vi "SP Stimulus Debuging Tool.vi"(5 "New Stimulus":T1={"Use Instrument Settings"=FALSE, "Blank Frequencies"=FALSE, "Sweep Type"=enum."Linear", "Sweep"={"Fstart"=500.0, "Fstop"=1500.0, "Units"=enum."MHz", "Points"=201}, "Power (dBm)"=999.0, "IFBW (Hz)"=-1.0, "Sweep Time (s)"=-1.0, "Calibration"={"State"=FALSE, "String"=""}} {"Sweep Time (s)" format="%.3g"}, 7 "Current Stimulus":T1={"Use Instrument Settings"=FALSE, "Blank Frequencies"=FALSE, "Sweep Type"=enum."Linear", "Sweep"={"Fstart"=500.0, "Fstop"=1500.0, "Units"=enum."MHz", "Points"=201}, "Power (dBm)"=999.0, "IFBW (Hz)"=-1.0, "Sweep Time (s)"=-1.0, "Calibration"={"State"=FALSE, "String"=""}} {"Sweep Time (s)" format="%.3g"}, 8 "Overall":bool, 9 "SweepTime":bool, 10 "IFBW":bool, 11 "Power":bool) -> ()   [LabVIEW 2011]
uses:
  TypeDefs/SP Stimulus Parameters.ctl
  TypeDefs/SP Frequency Units.ctl
  TypeDefs/SP Calibration State.ctl
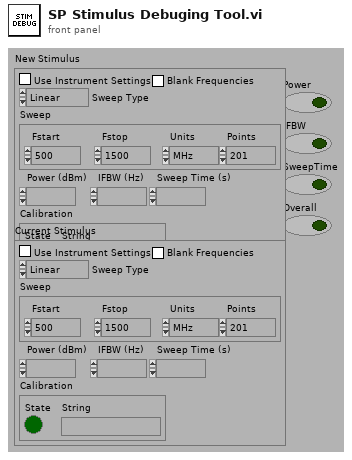
[diagram p1: front panel]
types:
  T1 = typedef "SP Stimulus Parameters.ctl" = cluster{"Use Instrument Settings":bool, "Blank Frequencies":bool, "Sweep Type":enum32{"Linear", "Logarithmic", "List", "Power", "CW"}, "Sweep":cluster{"Fstart":dbl, "Fstop":dbl, "Units":T2, "Points":i32}, "Power (dBm)":dbl, "IFBW (Hz)":dbl, "Sweep Time (s)":dbl, "Calibration":T3}
  T2 = typedef "SP Frequency Units.ctl" = enum16{"Hz", "kHz", "MHz", "GHz", "Points"}
  T3 = typedef "SP Calibration State.ctl" = cluster{"State":bool, "String":string}
  T4 = cluster{"Fstart":dbl, "Fstop":dbl, "Units":T2, "Points":i32}
  T5 = enum32{"Linear", "Logarithmic", "List", "Power", "CW"}
  T6 = enum32{"invalid app kind", "Development System", "Run Time System", "Student Edition", "Embedded LabVIEW", "Evaluation", "Custom"}
  T7 = enum16{"open", "replace", "create", "open or create", "replace or create", "replace or create with confirmation"}
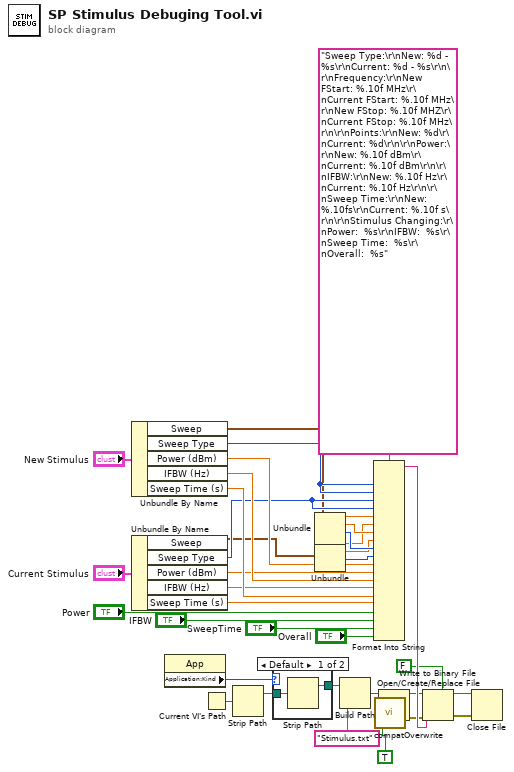
[diagram p0: block diagram]
diagram:
  n1 = Unbundle By Name("New Stimulus") -> ("Sweep"=w2:T4, "Sweep Type"=w13:T5, "Power (dBm)"=w12:dbl, "IFBW (Hz)"=w11:dbl, "Sweep Time (s)"=w10:dbl)
  n2 = Unbundle By Name("Current Stimulus") -> ("Sweep"=w1:T4, "Sweep Type"=w8:T5, "Power (dBm)"=w7:dbl, "IFBW (Hz)"=w6:dbl, "Sweep Time (s)"=w5:dbl)
  n3 = property class="App"() -> ("Application:Kind"=w23:T6)  [unwired: 2 in, 2 out]
  n4 = Current VI's Path() -> (path=w19:path)
  n5 = Strip Path(path=w19) -> (stripped path=w21:path)  [unwired: 1 out]
  n6 = case shown="Default" w23 {
    tunnel: w21 -> [w39 w40]
    tunnel: [w38 w40] -> w22
    frame Default {
      n7 = Strip Path(path=w39) -> (stripped path=w38:path)  [unwired: 1 out]
    }
    frame "Development System" {
    }
  }
  n8 = Unbundle(w2) -> ("Fstart"=w26:dbl, "Fstop"=w28:dbl, "Units"=w30:T2)  [unwired: 1 out]
  n9 = Unbundle(w1) -> ("Fstart"=w27:dbl, "Fstop"=w29:dbl, "Units"=w31:T2)  [unwired: 1 out]
  n10 = Build Path(base path=w22, name or relative path="Stimulus.txt") -> (appended path=w24:path)
  n11 = Format Into String(format string="Sweep Type:\r\nNew: %d - %s\r\nCurrent: %d - %s\r\n\r\nFrequency:\r\nNew FStart: %.10f MHz\r\nCurrent FStart: %.10f MHz\r\nNew FStop: %.10f MHZ\r\nCurrent FStop: %.10f MHz\r\n\r\nPoints:\r\nNew: %d\r\nCurrent: %d\r\n\r\nPower:\r\nNew: %.10f dBm\r\nCurrent: %.10f dBm\r\n\r\nIFBW:\r\nNew: %.10f Hz\r\nCurrent: %.10f Hz\r\n\r\nSweep Time:\r\nNew: %.10fs\r\nCurrent: %.10f s\r\n\r\nStimulus Changing:\r\nPower:  %s\r\nIFBW:  %s\r\nSweep Time:  %s\r\nOverall:  %s", w13, w13, w8, w8, w26, w27, w28, w29, w30, w31, w12, w7, w11, w6, w10, w5, "Power", "IFBW", "SweepTime", "Overall") -> (resulting string=w32:string)  [unwired: 2 in, 1 out]
  n12 = call <vilib>:"compatOverwrite.vi"("overwrite (F)"=TRUE) -> ("overwrite?"=w3:T7)
  n13 = Open/Create/Replace File(file path (use dialog)=w24, operation (0:open)=w3) -> (refnum out=w18:refnum<file>, error out=w15:errorcluster)  [unwired: 1 in, 4 out]
  n14 = Write to Binary File(file (use dialog)=w18, data=w32, error in=w15, 5:FALSE ("prepend array or string size? (T)")) -> (refnum out=w17:refnum<file>, error out=w16:errorcluster)  [unwired: 3 out]
  n15 = Close File(refnum=w17, error in=w16) -> ()  [unwired: 2 out]
